vi "Create Session Reservation.vi"(7 "reservation observer":refnum<class "IReservationObserver.lvclass">, 8 "error in (no error)":errorcluster, 9 "sessions":T1[](array[typedef]), 10 "pin or relay names":string[](array[string]), 11 "pin map context":T4) -> (0 "error out":errorcluster, 3 "session reservation out":refnum<class "Session Reservation.lvclass">)   [LabVIEW 2020, in "MeasurementLink Session Management.lvlib" / "Session Reservation.lvclass"]
uses:
  Session Reservation.lvclass
  Session Reservation.lvclass/Session Reservation.ctl
  MeasurementLink Instrument/IInstrument/IInstrument.lvclass
  MeasurementLink Session Management Client/RPC Messages/ni_measurementlink_sessionmanagement_v1_ChannelMapping.ctl
  MeasurementLink Session Management Client/MeasurementLink Session Management Client.lvlib
  MeasurementLink Session Management Client/RPC Messages/nidevice_grpc_Session.ctl
  MeasurementLink Session Management Client/RPC Messages/ni_measurementlink_sessionmanagement_v1_SessionInformation.ctl
  Session and Driver Info.ctl
  MeasurementLink Session Management Client/RPC Messages/ni_measurementlink_PinMapContext.ctl
  Connection Map/Connection Map.lvclass
  Data.ctl
  IReservationObserver/IReservationObserver.lvclass
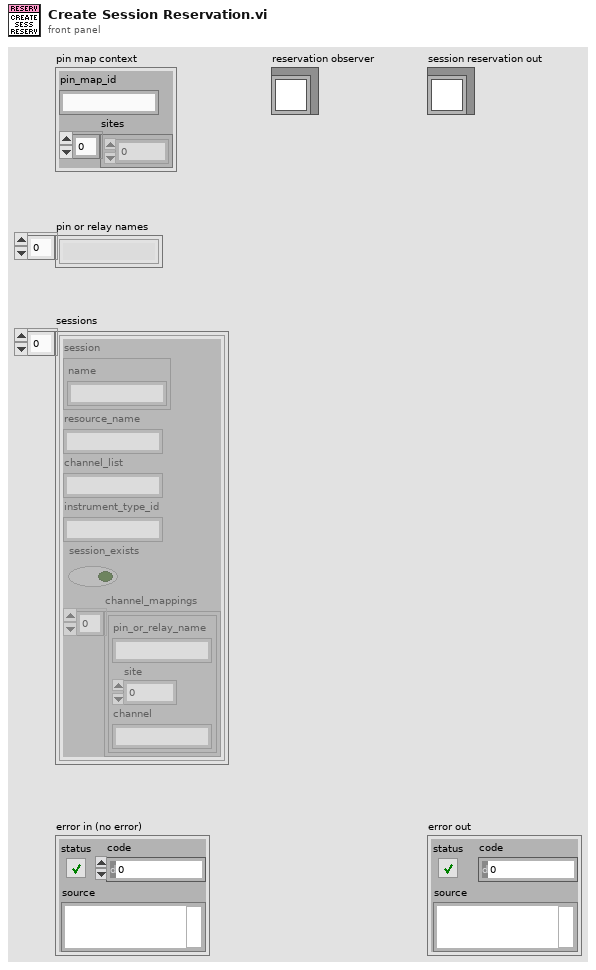
[diagram p1: front panel]
types:
  T1 = typedef "MeasurementLink Session Management Client.lvlib/ni_measurementlink_sessionmanagement_v1_SessionInformation.ctl" = cluster{"session":T2, "resource_name":string, "channel_list":string, "instrument_type_id":string, "session_exists":bool, "channel_mappings":T3[]}
  T2 = typedef "MeasurementLink Session Management Client.lvlib/nidevice_grpc_Session.ctl" = cluster{"name":string}
  T3 = typedef "MeasurementLink Session Management Client.lvlib/ni_measurementlink_sessionmanagement_v1_ChannelMapping.ctl" = cluster{"pin_or_relay_name":string, "site":i32, "channel":string}
  T4 = typedef "MeasurementLink Session Management Client.lvlib/ni_measurementlink_PinMapContext.ctl" = cluster{"pin_map_id":string, "sites":i32[]}
  T5 = typedef "MeasurementLink Session Management.lvlib/Session Reservation.lvclass/Data.ctl" = cluster{"session and driver infos":T6[], "pin or relay names":string[], "connection map":refnum<class "Connection Map.lvclass">, "pin map context":T4, "reservation observer":refnum<class "IReservationObserver.lvclass">, "dvr valid":bool}
  T6 = typedef "MeasurementLink Session Management.lvlib/Session Reservation.lvclass/Session and Driver Info.ctl" = cluster{"session info":T1, "session":variant, "instrument":refnum<class "IInstrument.lvclass">}
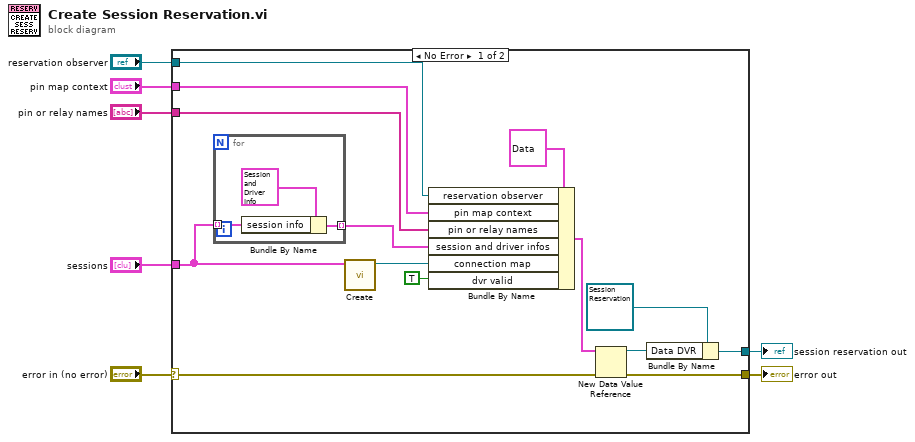
[diagram p0: block diagram]
diagram:
  n1 = case shown="No Error" "error in (no error)" {
    selector: "error in (no error)" -> [w11 w25]
    tunnel: [w15 w25] -> w7
    tunnel: [w14 _] -> w6
    tunnel: "sessions" -> [w10 _]
    tunnel: "pin map context" -> [w13 _]
    tunnel: "pin or relay names" -> [w12 _]
    tunnel: "reservation observer" -> [w9 _]
    frame No Error {
      n2 = for {
        tunnel: w10 -> [w24] mode=indexing
        tunnel: [w23] -> w21 mode=indexing
        n3 = Bundle By Name(cluster=T6 {"session info"={"session"={"name"=""}, "resource_name"="", "channel_list"="", "instrument_type_id"="", "session_exists"=FALSE, "channel_mappings"=[]}, "session"=variant, "instrument"=refnum} ("session and driver info"), "session info"=w24) -> (w23:T6)
      }
      n4 = call "Create.vi"("session info"=w10) -> ("connection map"=w20:refnum<class "Connection Map.lvclass">)  [unwired: 10 in]
      n5 = Bundle By Name(cluster=T5 {"session and driver infos"=[], "pin or relay names"=[], "connection map"=refnum, "pin map context"={"pin_map_id"="", "sites"=[]}, "reservation observer"=refnum, "dvr valid"=FALSE} ("session reservation data"), "reservation observer"=w9, "pin map context"=w13, "pin or relay names"=w12, "session and driver infos"=w21, "connection map"=w20, "dvr valid"=TRUE) -> (w17:T5)
      n6 = New Data Value Reference(data value=w17, error in=w11) -> (data value reference=w19:refnum<data-value>, error out=w15:errorcluster)
      n7 = Bundle By Name(cluster=refnum<class "Session Reservation.lvclass"> refnum ("session reservation"), "Data DVR"=w19) -> (w14:refnum<class "Session Reservation.lvclass">)
    }
    frame Error {
    }
  }
  "error out" <- w7
  "session reservation out" <- w6
